vi "ExtractStatusFromCOMbuffer.vi"(8 "error in (no error)":errorcluster, 11 "Input OPC data":string) -> (0 "error out":errorcluster, 2 "Valid Data":bool, 3 "GRIMM STATUS":i32[](array[numeric]))   [LabVIEW 2013]
doc: "Use this template to build a VI to use as a subVI."
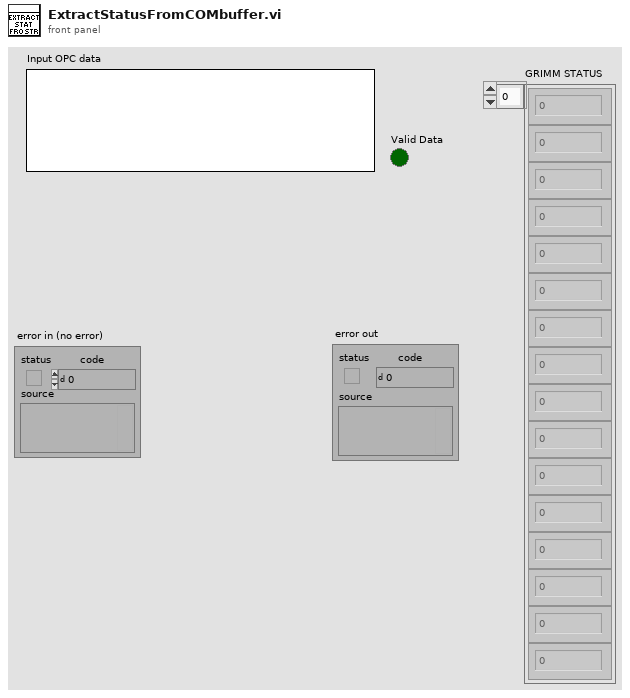
[diagram p1: front panel]
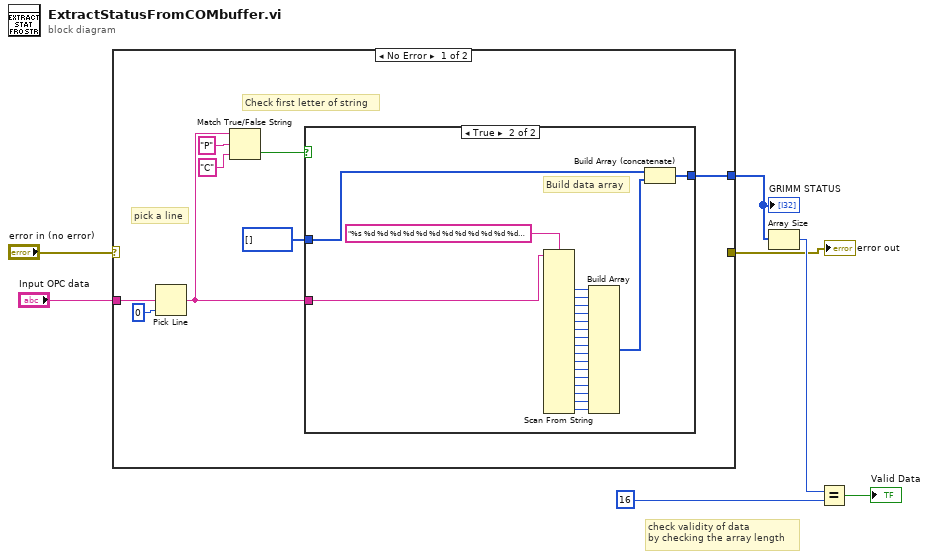
[diagram p0: block diagram]
diagram:
  # "check validity of data\nby checking the array length"
  n1 = case shown="No Error" "error in (no error)" {
    selector: "error in (no error)" -> [_ w38]
    tunnel: [_ w38] -> w1
    tunnel: "Input OPC data" -> [w15 _]
    tunnel: [w13 _] -> w2
    frame No Error {
      # "pick a line"
      # "Check first letter of string"
      n2 = Pick Line(multi-line string=w15, line index=0) -> (output string=w10:string)  [unwired: 1 in]
      n3 = Match True/False String(2:"C" ("false string"), 3:"P" ("true string"), 4:w10) -> (0:w8:bool)  [unwired: 1 out]
      n4 = case shown="True" w8 {
        tunnel: w10 -> [_ w29]
        tunnel: i32[] [] ("Output Number of Particles per 100 CC") -> [w16 w27]
        tunnel: [w16 w25] -> w13
        frame False {
        }
        frame True {
          # "Build data array"
          n5 = Scan From String(format string="%s %d %d %d %d %d %d %d %d %d %d %d %d %d %d %d %d", input string=w29) -> (output 2=w30:i32, output 3=w31:i32, output 4=w32:i32, output 5=w33:i32, output 6=w34:i32, output 7=w35:i32, output 8=w36:i32, output 9=w37:i32, output 10=w24:i32, output 11=w23:i32, output 12=w22:i32, output 13=w21:i32, output 14=w20:i32, output 15=w19:i32, output 16=w18:i32, output 17=w17:i32)  [unwired: 20 in, 3 out]
          n6 = Build Array(w30, w31, w32, w33, w34, w35, w36, w37, w24, w23, w22, w21, w20, w19, w18, w17) -> (w26:i32[])
          n7 = Build Array (concatenate)(w27, w26) -> (w25:i32[])
        }
      }
    }
    frame Error {
    }
  }
  "error out" <- w1
  "GRIMM STATUS" <- w2
  n8 = Array Size(array=w2) -> (size(s)=w5:i32)
  n9 = Equal?(x=w5, y=16) -> (x = y?=→"Valid Data":bool)
